vi "Grab_x64.vi"() -> ()   [LabVIEW 2015]
panel:
  out "Image":T1(plugin-control)
  in  "Snap Image":bool
  in  "stop":bool
  in  "ICImagingControl":refnum<k7>(container)
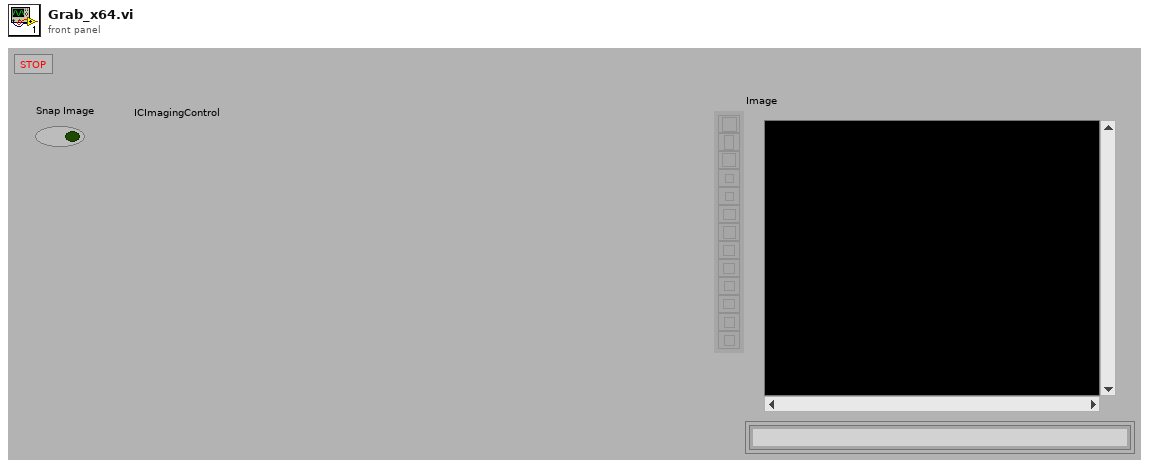
[diagram p1: front panel]
types:
  T1 = typedef "IMAQ Image.ctl" = refnum<image>
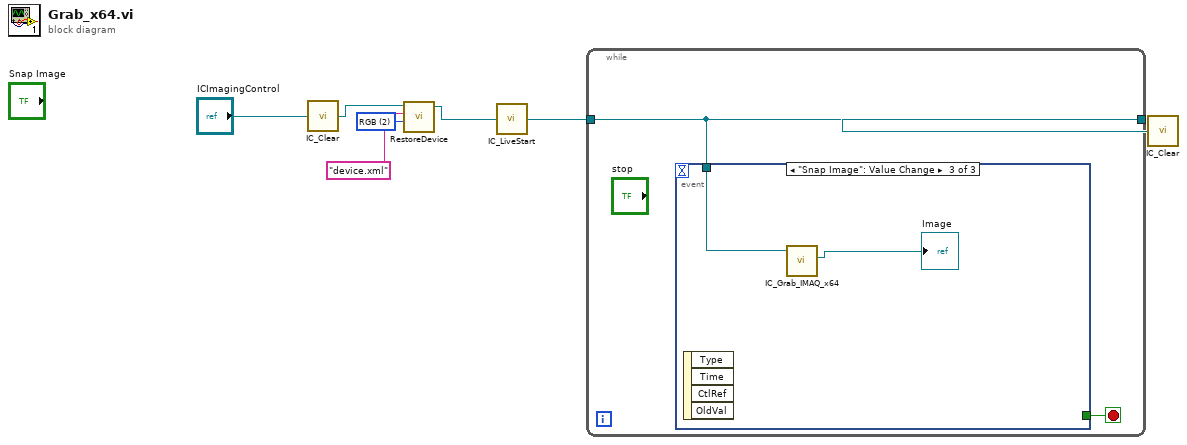
[diagram p0: block diagram]
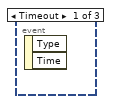
[diagram p2: hidden frame]
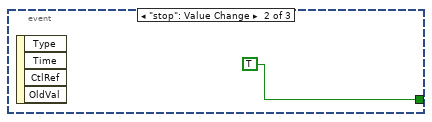
[diagram p3: hidden frame]
diagram:
  w1 = u16 2 items=["RGB"=2, "Y800"=5, "Y16"=11] ("Color modes")
  n1 = call "IC_Clear.vi"("ICImagingControl 2"="ICImagingControl") -> ("ICImagingControl"=w6:refnum<k7>)
  n2 = call "RestoreDevice.vi"("Color modes"=w1, "Filename"="device.xml", "ICImagingControl"=w6) -> ("ICImagingControl 2"=w5:refnum<k7>)  [unwired: 1 in, 2 out]
  n3 = call "IC_LiveStart.vi"("ICImagingControl 3"=w5) -> ("ICImagingControl 2"=w3:refnum<k7>)
  n4 = while {
    tunnel: [w8] -> w4
    tunnel: w3 -> [w8]
    stop <- w9 stop-if-true
    n5 = event shown="[2] \"Snap Image\": Value Change" {
      selector: _ -> [_ _ _]
      dyn-events: _ -> [_ _ _]
      timeout: _ -> [_ _ _]
      tunnel: [_ TRUE _] -> w9
      tunnel: w8 -> [_ _ w12]
      event Timeout {
        n6 = event-data() -> ()  [unwired: 1 in, 2 out]
      }
      event "stop": Value Change {
        n7 = event-data() -> ()  [unwired: 1 in, 4 out]
      }
      event "Snap Image": Value Change {
        n8 = event-data() -> ()  [unwired: 1 in, 4 out]
        n9 = call "IC_Grab_IMAQ_x64.vi"("ICImagingControl In"=w12) -> ("Image Out"=→"Image":T1)  [unwired: 2 in, 3 out]
      }
    }
  }
  n10 = call "IC_Clear.vi"("ICImagingControl 2"=w4) -> ()  [unwired: 1 out]
